vi "TCPRouter ClientAPI Example 6.vi"() -> ()   [LabVIEW 2020]
uses:
  _addons/TCP-Router/ClientAPI/Def-TCP-Router Status Data.ctl
  <userlib>/_NEVSTOP/Communicable State Machine(CSM)/AdvanceAPI/CSM - Broadcast Message Type.ctl
  40172a79-c7d9-4584-8019-dfe908fc4a6d.vi
  b3b63605-1016-4be4-a788-12e3256b011c.vi
  7e38bf89-2462-47fa-b6f6-5b46729ec3b2.vi
  _addons/TCP-Router/ClientAPI/TcpRouter-Client.lvclass
  <userlib>/_NEVSTOP/Communicable State Machine(CSM)/Communicable State Machine.lvlib
panel:
  out "Waveform Chart":waveform(i16)[](graph)
  out "error out 2":errorcluster
  out "error out":errorcluster
  out "element 2":T1
  out "# elements in queue 2":i32
  out "# elements in queue":i32
  out "current time":timestamp
  out "element":T1
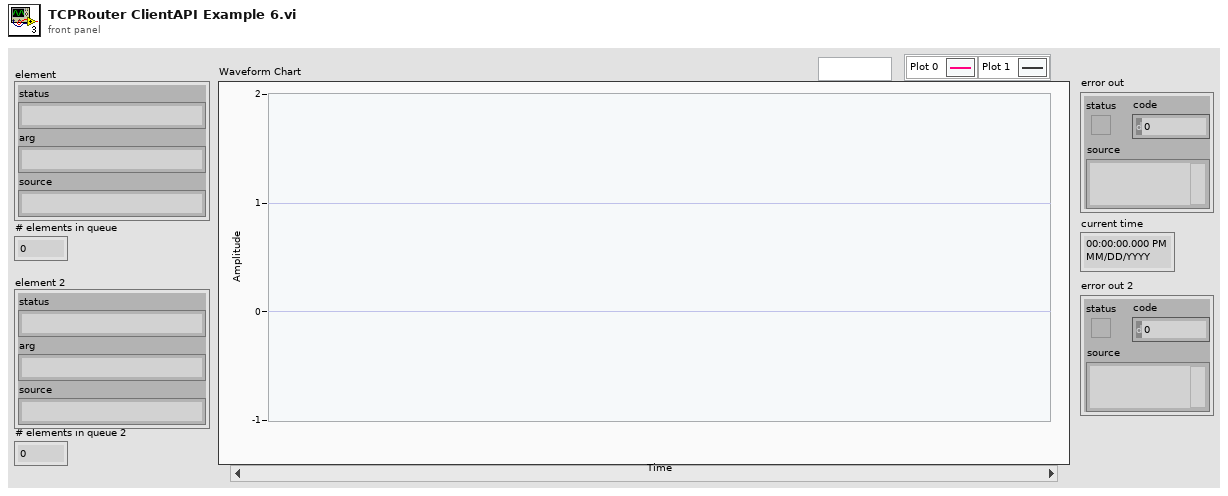
[diagram p1: front panel]
types:
  T1 = typedef "CSM-TCP-Router.lvlib/TcpRouter-Client.lvclass/Def-TCP-Router Status Data.ctl" = cluster{"status":string, "arg":string, "source":string}
  T2 = typedef "Communicable State Machine.lvlib/CSM - Broadcast Message Type.ctl" = enum16{"<Null>", "Status", "Interrupt"}
  T3 = cluster{"IP Address":string, "Port":u16, "ConnectTMO":i32}
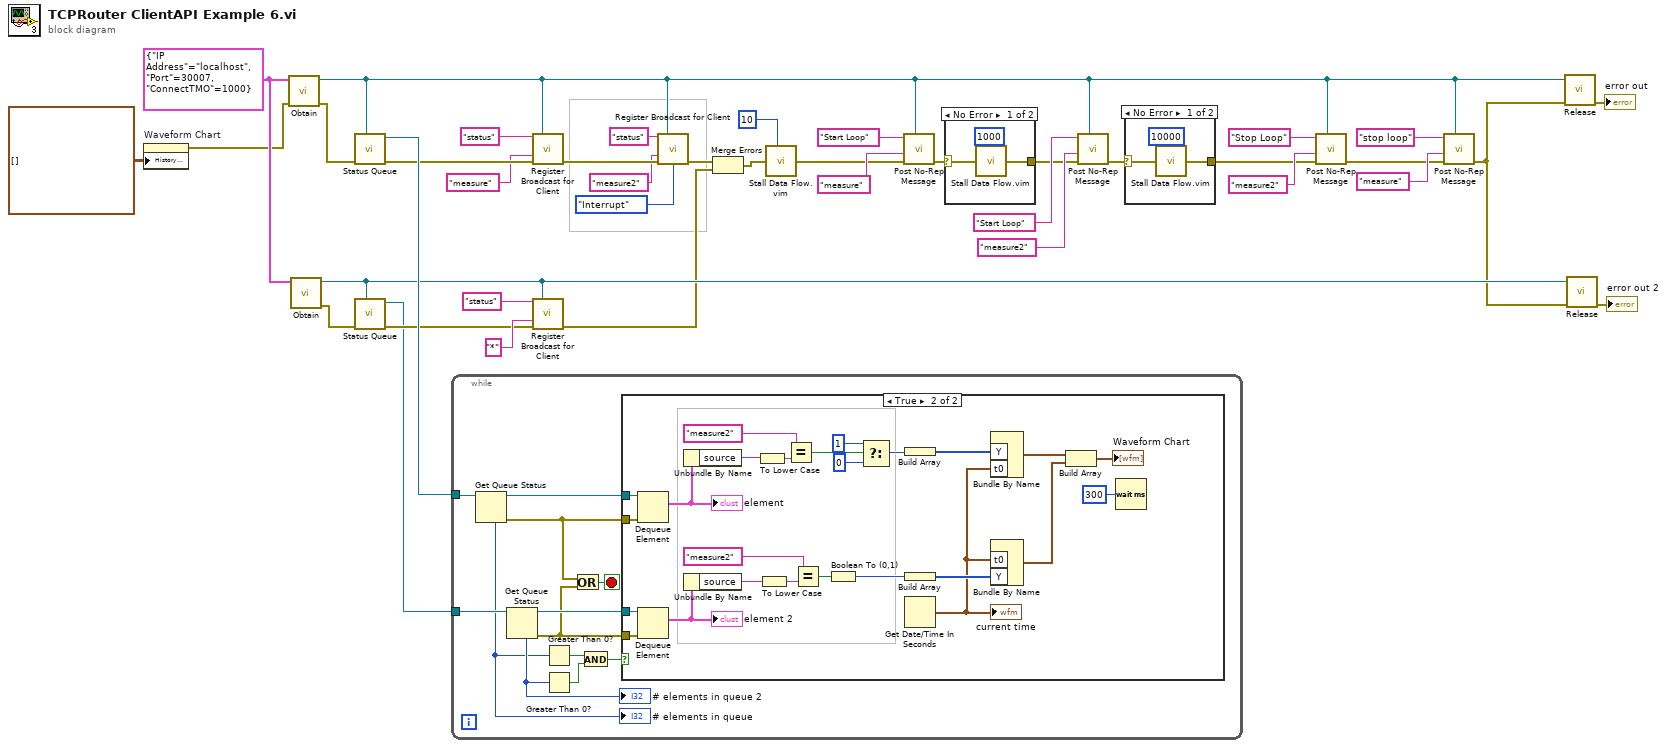
[diagram p0: block diagram]
diagram:
  w27 = T3 {"IP Address"="localhost", "Port"=30007, "ConnectTMO"=1000} ("Connection")
  n1 = property on="Waveform Chart" class="WFChart (strict)"("History Data"=waveform(i16)[][] []) -> (error out=w1:errorcluster)  [unwired: 2 in, 1 out]
  n2 = call "Obtain.vi"("error in (no error)"=w1, "Connection"=w27) -> ("error out"=w35:errorcluster, "TcpRouter-Client out"=w6:refnum<class "TcpRouter-Client.lvclass">)  [unwired: 8 in]
  n3 = call "Obtain.vi"("Connection"=w27) -> ("error out"=w28:errorcluster, "TcpRouter-Client out"=w34:refnum<class "TcpRouter-Client.lvclass">)  [unwired: 9 in]
  n4 = call "Status Queue.vi"("TcpRouter-Client in"=w6, "error in (no error)"=w35) -> ("error out"=w26:errorcluster, "StatusQueue"=w36:refnum<queue>)  [unwired: 8 in]
  n5 = call "Status Queue.vi"("TcpRouter-Client in"=w34, "error in (no error)"=w28) -> ("error out"=w29:errorcluster, "StatusQueue"=w3:refnum<queue>)  [unwired: 8 in]
  n6 = while {
    tunnel: w36 -> [w52]
    tunnel: w3 -> [w49]
    stop <- w41 stop-if-true
    n7 = Get Queue Status(queue=w52) -> (queue out=w51:refnum<queue>, error out=w43:errorcluster, # elements in queue=w44:i32)  [unwired: 2 in, 5 out]
    "# elements in queue" <- w44
    n8 = Get Queue Status(queue=w49) -> (queue out=w50:refnum<queue>, error out=w42:errorcluster, # elements in queue=w48:i32)  [unwired: 2 in, 5 out]
    "# elements in queue 2" <- w48
    n9 = Greater Than 0?(x=w44) -> (x > 0?=w47:bool)
    n10 = Greater Than 0?(x=w48) -> (x > 0?=w46:bool)
    n11 = Or(x=w43, y=w42) -> (x .or. y?=w41:bool)
    n12 = And(x=w47, y=w46) -> (x .and. y?=w45:bool)
    n13 = case shown="True" w45 {
      tunnel: w51 -> [_ w77]
      tunnel: w43 -> [_ w75]
      tunnel: w42 -> [_ w74]
      tunnel: w50 -> [_ w72]
      frame False {
      }
      frame True {
        n14 = Dequeue Element(queue=w77, error in (no error)=w75) -> (element=w76:T1)  [unwired: 1 in, 3 out]
        "element" <- w76
        n15 = Dequeue Element(queue=w72, error in (no error)=w74) -> (element=w73:T1)  [unwired: 1 in, 3 out]
        "element 2" <- w73
        n16 = Unbundle By Name(w76) -> ("source"=w70:string)
        n17 = Unbundle By Name(w73) -> ("source"=w67:string)
        n18 = To Lower Case(string=w70) -> (all lower case string=w69:string)
        n19 = To Lower Case(string=w67) -> (all lower case string=w65:string)
        n20 = Equal?(x="measure2" ("Source CSM Name (* as Default)"), y=w69) -> (x = y?=w57:bool)
        n21 = Equal?(x="measure2" ("Source CSM Name (* as Default)"), y=w65) -> (x = y?=w66:bool)
        n22 = Boolean To (0,1)(Boolean=w66) -> (0, 1=w62:i16)
        n23 = Select(t=i16 1 ("0, 1"), s=w57, f=i16 0) -> (s? t:f=w55:i16)
        n24 = Build Array(w55) -> (w64:i16[])
        n25 = Build Array(w62) -> (w63:i16[])
        n26 = Get Date/Time In Seconds() -> (seconds since 1Jan1904=w58:timestamp)
        "current time" <- w58
        n27 = Bundle By Name("Y"=w64, "t0"=w58) -> (w61:waveform(i16))  [unwired: 1 in]
        n28 = Bundle By Name("t0"=w58, "Y"=w63) -> (w60:waveform(i16))  [unwired: 1 in]
        n29 = Build Array(w61, w60) -> (→"Waveform Chart":waveform(i16)[])
        n30 = Wait (ms)(milliseconds to wait=u32 300) -> ()  [unwired: 1 out]
      }
    }
  }
  n31 = call "Register Broadcast for Client.vi"("Status"="status" ("CSM Name"), "TcpRouter-Client in"=w6, "CSM Name"="measure" ("Source CSM Name (* as Default)"), "error in (no error)"=w26) -> ("error out"=w20:errorcluster)  [unwired: 10 in, 1 out]
  n32 = call "Register Broadcast for Client.vi"("Status"="status" ("CSM Name"), "TcpRouter-Client in"=w34, "CSM Name"="*" ("Source CSM Name (* as Default)"), "error in (no error)"=w29) -> ("error out"=w13:errorcluster)  [unwired: 10 in, 1 out]
  n33 = call "Register Broadcast for Client.vi"("Status"="status", "TcpRouter-Client in"=w6, "CSM Name"="measure2" ("Source CSM Name (* as Default)"), "error in (no error)"=w20, "Priority (No Change)"=CSM_-_Broadcast_Message_Type."Interrupt") -> ("error out"=w21:errorcluster)  [unwired: 9 in, 1 out]
  n34 = Merge Errors(w21, w13) -> (w16:errorcluster)
  n35 = call "Stall Data Flow.vim"("value in"=w16, "milliseconds to wait"=u32 10) -> ("value out"=w5:errorcluster)  [unwired: 1 out]
  n36 = call "Post No-Rep Message.vi"("TcpRouter-Client in"=w6, "error in (no error)"=w5, "Target Module"="measure", "State"="Start Loop") -> ("error out"=w12:errorcluster)  [unwired: 7 in]
  n37 = case shown="No Error" w12 {
    selector: w12 -> [w78 w81]
    tunnel: [w80 w81] -> w11
    frame No Error {
      n38 = call "Stall Data Flow.vim"("value in"=w78, "milliseconds to wait"=u32 1000) -> ("value out"=w80:errorcluster)  [unwired: 1 out]
    }
    frame Error {
    }
  }
  n39 = call "Post No-Rep Message.vi"("TcpRouter-Client in"=w6, "error in (no error)"=w11, "Target Module"="measure2", "State"="Start Loop") -> ("error out"=w10:errorcluster)  [unwired: 7 in]
  n40 = case shown="No Error" w10 {
    selector: w10 -> [w82 w85]
    tunnel: [w84 w85] -> w9
    frame No Error {
      n41 = call "Stall Data Flow.vim"("value in"=w82, "milliseconds to wait"=u32 10000) -> ("value out"=w84:errorcluster)  [unwired: 1 out]
    }
    frame Error {
    }
  }
  n42 = call "Post No-Rep Message.vi"("TcpRouter-Client in"=w6, "error in (no error)"=w9, "Target Module"="measure2", "State"="Stop Loop") -> ("error out"=w8:errorcluster)  [unwired: 7 in]
  n43 = call "Post No-Rep Message.vi"("TcpRouter-Client in"=w6, "error in (no error)"=w8, "Target Module"="measure", "State"="stop loop") -> ("error out"=w7:errorcluster)  [unwired: 7 in]
  n44 = call "Release.vi"("error in (no error)"=w7, "TcpRouter-Client in"=w6) -> ("error out"=→"error out":errorcluster)  [unwired: 9 in]
  n45 = call "Release.vi"("error in (no error)"=w7, "TcpRouter-Client in"=w34) -> ("error out"=→"error out 2":errorcluster)  [unwired: 9 in]
